vi "Time Format.vi"(11 "time stamp":timestamp) -> (0 "concatenated string":string)   [LabVIEW 2018]
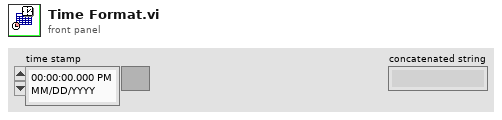
[diagram p1: front panel]
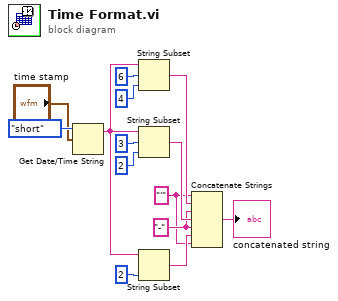
[diagram p0: block diagram]
diagram:
  w2 = "'" ("string")
  w5 = "-" ("string")
  n1 = Get Date/Time String(date format (0)=enum16{"short", "long", "abbreviated"}."short", seconds (now)="time stamp") -> (date string=w10:string)  [unwired: 1 in, 1 out]
  n2 = String Subset(string=w10, offset (0)=6, length (rest)=4 ("length (rest)")) -> (substring=w7:string)
  n3 = String Subset(string=w10, offset (0)=3, length (rest)=2 ("length (rest)")) -> (substring=w6:string)
  n4 = String Subset(string=w10, length (rest)=2 ("length (rest)")) -> (substring=w4:string)  [unwired: 1 in]
  n5 = Concatenate Strings(w2, w7, w5, w6, w5, w4, w2) -> (→"concatenated string":string)
